vi "UnInstallGRPCPackages.vi"() -> (0 "error out":errorcluster)   [LabVIEW 2019]
uses:
  <vilib>/JKI/VIPM API/VIPM API_vipm_api.lvlib
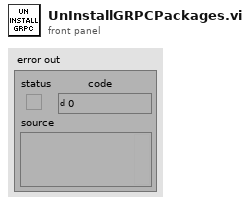
[diagram p1: front panel]
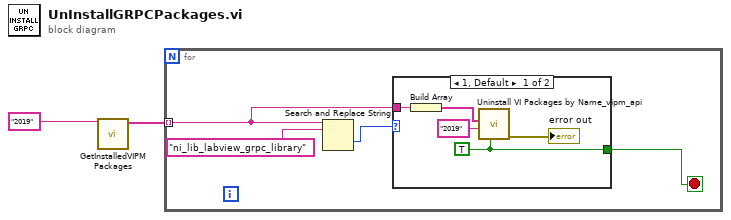
[diagram p0: block diagram]
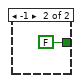
[diagram p2: hidden frame]
diagram:
  n1 = call "GetInstalledVIPMPackages.vi"("LabVIEW Version"="2019") -> ("Array"=w1:string[])  [unwired: 10 in]
  n2 = for {
    tunnel: w1 -> [w3] mode=indexing
    stop <- w4 stop-if-true
    n3 = Search and Replace String(input string=w3, search string="ni_lib_labview_grpc_library") -> (offset past replacement=w5:i32)  [unwired: 6 in, 3 out]
    n4 = case shown="1, Default" w5 {
      tunnel: [w9 FALSE ("quiet? (T)")] -> w4
      tunnel: w3 -> [w8 _]
      frame 1, Default {
        w9 = TRUE ("quiet? (T)")
        n5 = Build Array(w8) -> (w7:string[])
        n6 = call <vilib>:"Uninstall VI Packages by Name_vipm_api.vi"("quiet? (T)"=w9, "LabVIEW Version"="2019", "Package Names to Uninstall []"=w7) -> ("error out"=→"error out":errorcluster)  [unwired: 8 in]
      }
      frame -1 {
      }
    }
  }
